vi "Pendulo_Triple.vi"() -> ()   [LabVIEW 2016]
panel:
  out "XY Graph":cluster{dbl[], dbl[]}(graph)
  in  "L3":dbl(slide) scale=0.0..3.0
  in  "L2":dbl(slide) scale=0.0..3.0
  in  "L1":dbl(slide) scale=0.0..3.0
  in  "T3":dbl(knob)
  in  "T2":dbl(knob)
  in  "T1":dbl(knob)
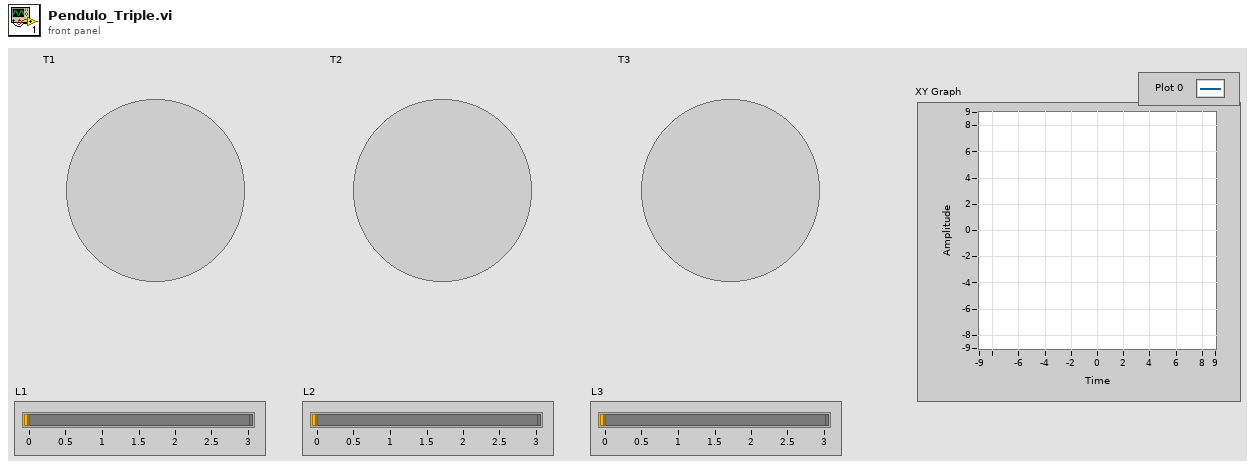
[diagram p1: front panel]
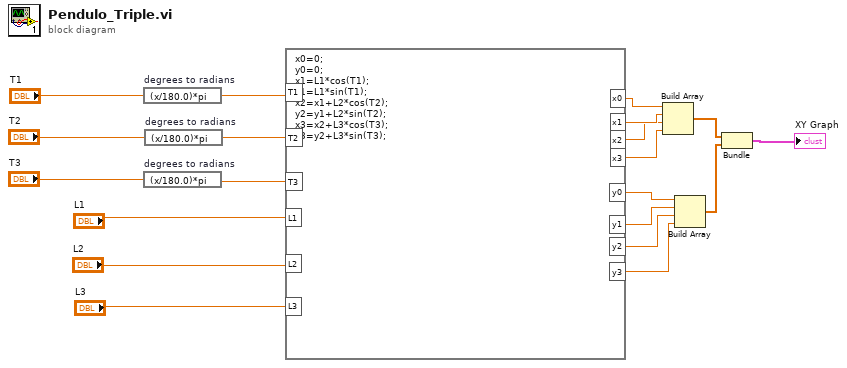
[diagram p0: block diagram]
diagram:
  n1 = expression code="(x/180.0)*pi" "degrees to radians"("T1") -> (w17:dbl)
  n2 = expression code="(x/180.0)*pi" "degrees to radians"("T3") -> (w6:dbl)
  n3 = expression code="(x/180.0)*pi" "degrees to radians"("T2") -> (w5:dbl)
  n4 = formula code="x0=0;\ny0=0;\nx1=L1*cos(T1);\ny1=L1*sin(T1);\nx2=x1+L2*cos(T2);\ny2=y1+L2*sin(T2);\nx3=x2+L3*cos(T3);\ny3=y2+L3*sin(T3);"("T1"=w17, "L1"="L1", "T2"=w5, "T3"=w6, "L2"="L2", "L3"="L3") -> ("x0"=w15:dbl, "x1"=w14:dbl, "y0"=w13:dbl, "y1"=w12:dbl, "x2"=w2:dbl, "x3"=w1:dbl, "y2"=w4:dbl, "y3"=w3:dbl)
  n5 = Build Array(w15, w14, w2, w1) -> (w11:dbl[])
  n6 = Build Array(w13, w12, w4, w3) -> (w10:dbl[])
  n7 = Bundle(w11, w10) -> (→"XY Graph":cluster{dbl[], dbl[]})  [unwired: 1 in]
